vi "draw.vi"(0 "reference":refnum<class "ChoiceNode.lvclass">, 1 "graphics":refnum<class "Graphics.lvclass">, 5 "error in (no error)":errorcluster) -> (14 "reference out":refnum<class "ChoiceNode.lvclass">, 19 "error out":errorcluster)   [LabVIEW 2020, in "ChoiceNode.lvclass"]
doc: "public void draw(Graphics2D g2, Point2D p, Point2D q)"
uses:
  <resource>/Framework/Providers/Open_GDS/UML/ChoiceNode_class/ChoiceNode.lvclass
  C:/Program Files (x86)/National Instruments/LabVIEW 2020/resource/Framework/Providers/Open_GDS/UML/RectangularNode_class/RectangularNode.lvclass
  <resource>/Framework/Providers/Open_GDS/UML/Graphics_class/Graphics.lvclass
  <resource>/Framework/Providers/Open_GDS/UML/General/Point/Point Point2D.ctl
  <resource>/Framework/Providers/Open_GDS/UML/UMLEditor/UMLEditor_StoredColors.ctl
  <resource>/Framework/Providers/Open_GDS/UML/MultiLineString_class/MultiLineString.lvclass
  <resource>/Framework/Providers/Open_GDS/UML/RectangularNode_class/RectangularNode.lvclass
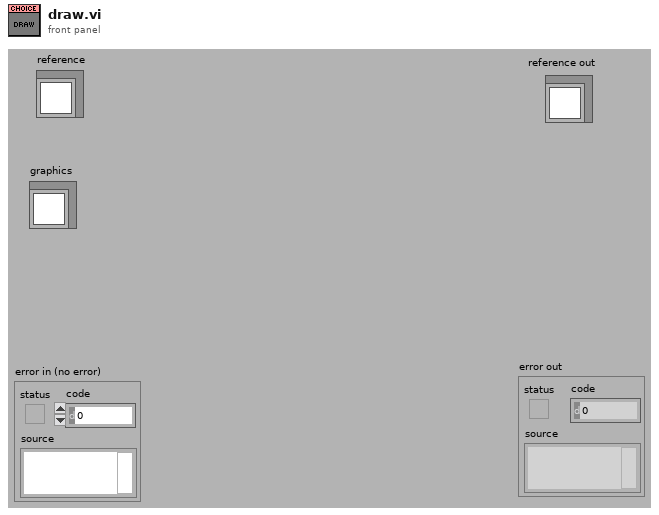
[diagram p1: front panel]
types:
  T1 = typedef "UMLEditor_StoredColors.ctl" = enum16{"ClassBackgroudColor", "ClassBackgroudColorWithClassPath", "ClassBackgroudColorForApplicationVIStereotype", "ClassBackgroudColorForTypeStereotype", "StateBackgroudColor"}
  T2 = typedef "Point Point2D.ctl" = cluster{"x":dbl, "y":dbl}
  T3 = typedef "ChoiceNode.lvclass/ObjectAttributes.ctl" = cluster{"Text":refnum<class "MultiLineString.lvclass">, "DEFAULT_WIDTH":i32, "DEFAULT_HEIGHT":i32}
  T4 = typedef "RectangularNode.lvclass/ObjectAttributes.ctl" = cluster{"bounds":T5}
  T5 = typedef "Rectangle Rectangle2D.ctl" = cluster{"x":dbl, "y":dbl, "width":dbl, "height":dbl}
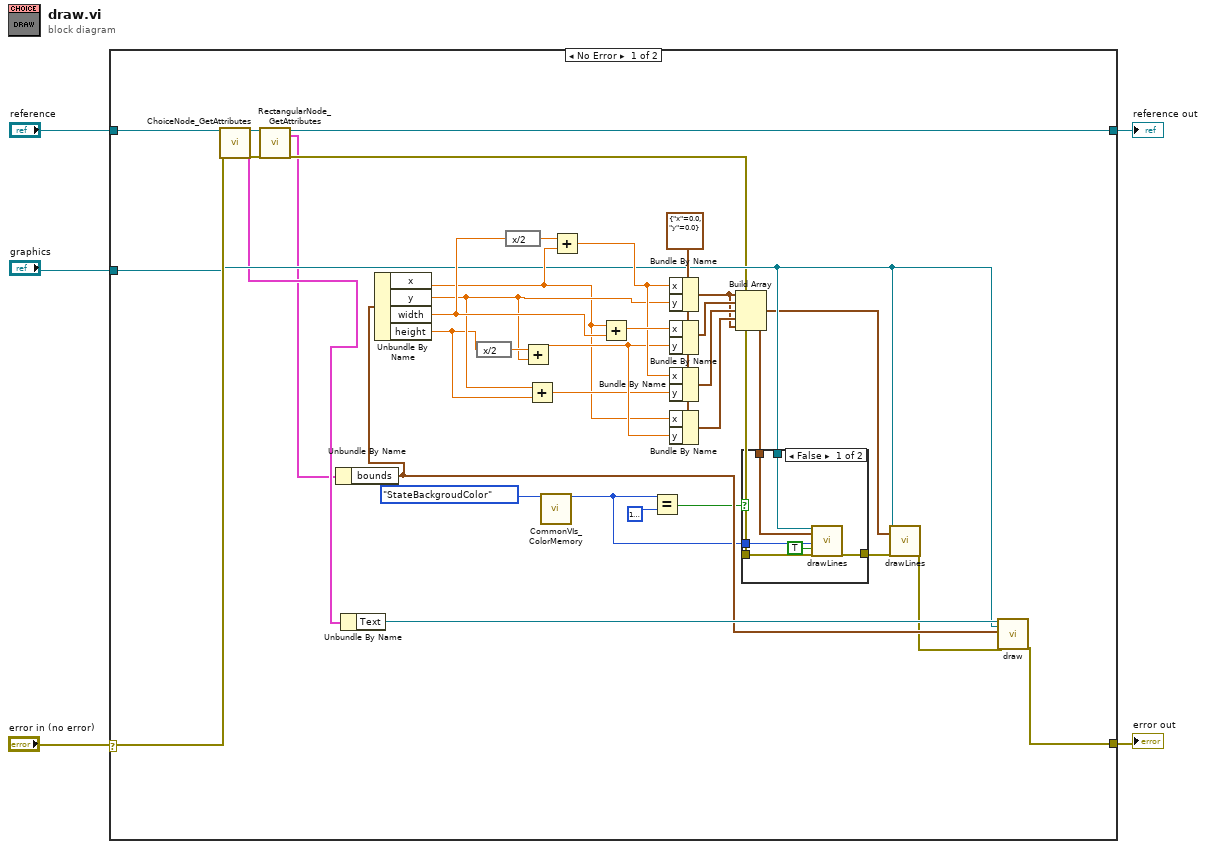
[diagram p0: block diagram]
diagram:
  n1 = case shown="No Error" "error in (no error)" {
    selector: "error in (no error)" -> [w35 w47]
    tunnel: "reference" -> [w39 w48]
    tunnel: [w34 w47] -> w4
    tunnel: [w7 w48] -> w3
    tunnel: "graphics" -> [w15 _]
    frame No Error {
      w29 = T2 {"x"=0.0, "y"=0.0} ("point2D")
      n2 = call <resource>:"ChoiceNode_GetAttributes.vi"("reference in"=w39, "error in (no error)"=w35) -> ("reference out"=w10:refnum<class "ChoiceNode.lvclass">, "Data"=w11:T3, "error out"=w9:errorcluster)  [unwired: 1 in, 14 out]
      n3 = call <resource>:"RectangularNode_GetAttributes.vi"("reference in"=w10, "error in (no error)"=w9) -> ("reference out"=w7:refnum<class "ChoiceNode.lvclass">, "Data"=w6:T4, "error out"=w8:errorcluster)  [unwired: 14 in, 1 out]
      n4 = Unbundle By Name(w6) -> ("bounds"=w20:T5)
      n5 = Unbundle By Name(w11) -> ("Text"=w38:refnum<class "MultiLineString.lvclass">)
      n6 = Unbundle By Name(w20) -> ("x"=w23:dbl, "y"=w26:dbl, "width"=w32:dbl, "height"=w25:dbl)
      n7 = expression code="x/2"(w25) -> (w30:dbl)
      n8 = expression code="x/2"(w32) -> (w31:dbl)
      n9 = Add(x=w30, y=w26) -> (x+y=w27:dbl)
      n10 = Add(x=w26, y=w25) -> (x+y=w24:dbl)
      n11 = call <resource>:"CommonVIs_ColorMemory.vi"("ColorName"=UMLEditor_StoredColors."StateBackgroudColor" ("UMLPathes")) -> ("Color Out"=w19:u32)  [unwired: 3 in, 15 out]
      n12 = Add(x=w31, y=w23) -> (x+y=w28:dbl)
      n13 = Add(x=w23, y=w32) -> (x+y=w37:dbl)
      n14 = Equal?(x=w19, y=u32 16777216) -> (x = y?=w17:bool)
      n15 = Bundle By Name(cluster=w29, "x"=w28, "y"=w26) -> (w13:T2)
      n16 = Bundle By Name(cluster=w29, "x"=w37, "y"=w27) -> (w36:T2)
      n17 = Bundle By Name(cluster=w29, "x"=w28, "y"=w24) -> (w22:T2)
      n18 = Bundle By Name(cluster=w29, "x"=w23, "y"=w27) -> (w21:T2)
      n19 = Build Array(w13, w36, w22, w21, w13) -> (w12:T2[])
      n20 = case shown="False" w17 {
        tunnel: [w45 w46] -> w16
        tunnel: w12 -> [w44 _]
        tunnel: w15 -> [w43 _]
        tunnel: w8 -> [w41 w46]
        tunnel: w19 -> [w40 _]
        frame False {
          n21 = call <resource>:"drawLines.vi"("reference"=w43, "points"=w44, "color(if not used=default color)"=w40, "fill?(F)"=TRUE, "error in (no error)"=w41) -> ("error out"=w45:errorcluster)  [unwired: 2 in, 12 out]
        }
        frame True {
        }
      }
      n22 = call <resource>:"drawLines.vi"("reference"=w15, "points"=w12, "error in (no error)"=w16) -> ("error out"=w14:errorcluster)  [unwired: 4 in, 12 out]
      n23 = call-dynamic "draw.vi"("reference"=w38, "graphics"=w15, "bounds"=w20, "error in (no error)"=w14) -> ("error out"=w34:errorcluster)  [unwired: 14 in, 1 out]
    }
    frame Error {
    }
  }
  "reference out" <- w3
  "error out" <- w4
